vi "Handle Endpoint Configuration Change.vi"(7 "Array in":refnum<vi>, 8 "error in (no error)":errorcluster, 9 "NewVal":T2[](array[typedef]), 10 "OldVal":T2[](array[typedef]), 11 "Endpoint Configuration Section Ref in":T1 format="%.0x") -> (0 "error out":errorcluster, 3 "Endpoint Configuration Section Ref out":T1 format="%.0x")   [LabVIEW 2017, in "SLSC Switch System Explorer.lvlib"]
uses:
  SLSC Switch System Explorer.lvlib
  Channel.ctl
  Channel Type.ctl
  <vilib>/NI Veristand/Custom Device API/Custom Device Item Ref.ctl
  Scripting/SLSC Switch Scripting.lvlib
  <vilib>/NI Veristand/Custom Device API/Custom Device API.lvlib
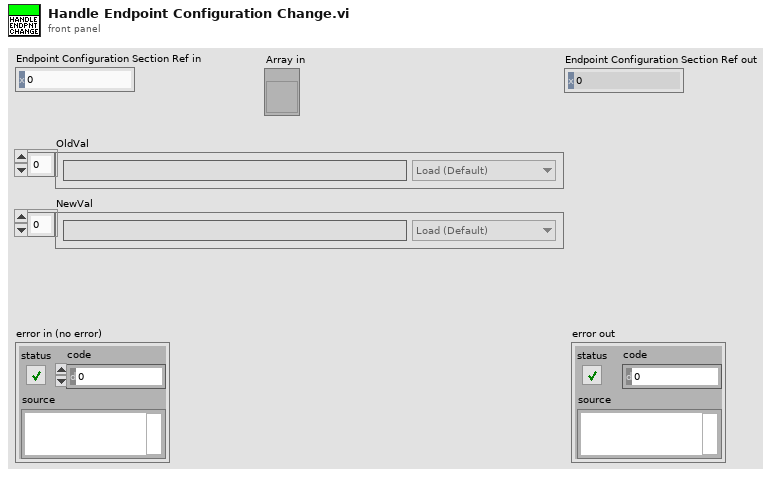
[diagram p1: front panel]
types:
  T1 = typedef "Custom Device API.lvlib/Custom Device Item Ref.ctl" = u64
  T2 = typedef "SLSC Switch System Explorer.lvlib/Channel.ctl" = cluster{"Endpoint":string, "Configuration":T3}
  T3 = typedef "SLSC Switch System Explorer.lvlib/Channel Type.ctl" = enum16{"Load (Default)", "Source", "Configuration"}
  T4 = typedef "SLSC Switch Shared.lvlib/Endpoint Configuration Cluster.ctl" = cluster{"Endpoint":string, "Configuration":T5}
  T5 = typedef "SLSC Switch Shared.lvlib/Endpoint Configuration Enum.ctl" = enum16{"Load", "Source", "Configuration"}
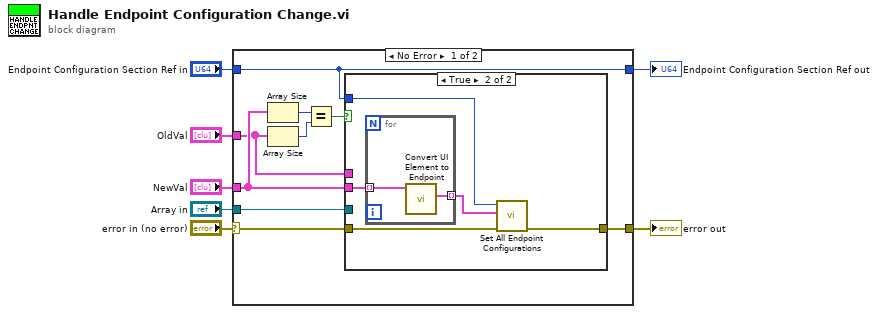
[diagram p0: block diagram]
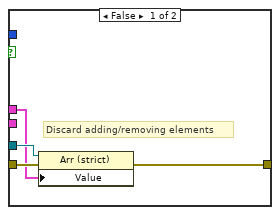
[diagram p2: hidden frame]
diagram:
  n1 = case shown="No Error" "error in (no error)" {
    selector: "error in (no error)" -> [w12 w28]
    tunnel: "NewVal" -> [w16 _]
    tunnel: "OldVal" -> [w15 _]
    tunnel: "Array in" -> [w14 _]
    tunnel: "Endpoint Configuration Section Ref in" -> [w8 w29]
    tunnel: [w13 w28] -> w3
    tunnel: [w8 w29] -> w1
    frame No Error {
      n2 = Array Size(array=w16) -> (size(s)=w9:i32)
      n3 = Array Size(array=w15) -> (size(s)=w10:i32)
      n4 = Equal?(x=w9, y=w10) -> (x = y?=w11:bool)
      n5 = case shown="True" w11 {
        tunnel: w12 -> [w20 w25]
        tunnel: [w19 w21] -> w13
        tunnel: w8 -> [_ w24]
        tunnel: w14 -> [w18 _]
        tunnel: w15 -> [w17 _]
        tunnel: w16 -> [_ w22]
        frame False {
          # "Discard adding/removing elements"
          n6 = property class="Arr (strict)"(reference=w18, error in=w20, "Value"=w17) -> (error out=w19:errorcluster)  [unwired: 1 out]
        }
        frame True {
          n7 = for {
            tunnel: [w27] -> w23 mode=indexing
            tunnel: w22 -> [w26] mode=indexing
            n8 = call "Convert UI Element to Endpoint.vi"("Channel"=w26) -> ("Connection"=w27:T4)  [unwired: 9 in, 1 out]
          }
          n9 = call "Set All Endpoint Configurations.vi"("error in (no error)"=w25, "All Endpoint Configurations"=w23, "Endpoint Configuration Section Ref in"=w24) -> ("error out"=w21:errorcluster)  [unwired: 7 in, 1 out]
        }
      }
    }
    frame Error {
    }
  }
  "error out" <- w3
  "Endpoint Configuration Section Ref out" <- w1
